vi "VI Tree.vi"   [LabVIEW 2012, in "Phidget Temperature Sensor.lvlib"]
doc: "${TemperatureSensor:VITreeHeader}"
uses:
  <instrlib>/Phidgets/Phidget Temperature Sensor/Phidget Temperature Sensor.lvlib
  <instrlib>/Phidgets/Phidget Temperature Sensor/Public/TemperatureSensorStart.vi
  <instrlib>/Phidgets/Phidget Temperature Sensor/Public/TemperatureSensorOpen.vi
  <instrlib>/Phidgets/Phidget Temperature Sensor/Public/TemperatureSensorClose.vi
panel:
  # "(c) 2015 Phidgets Inc..  ALL RIGHTS RESERVED."
  # "SEE DIAGRAM\nFOR VI TREE."
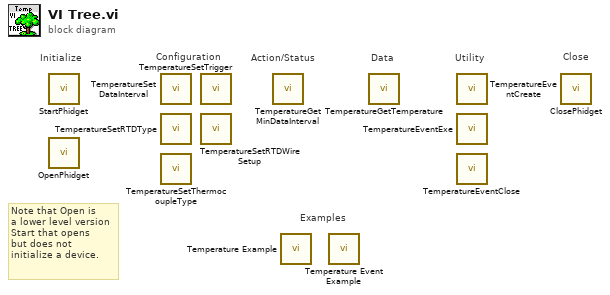
[diagram p0: block diagram]
diagram:
  # "Note that Open is\na lower level version\nStart that opens\nbut does not \ninitialize a device."
  # "Examples"
  # "Configuration"
  # "Utility"
  # "Data"
  # "Action/Status"
  # "Close"
  # "Initialize"
  n1 = call-poly <instrlib>:"StartPhidget.vi"() -> ()  [unwired: 12 in, 4 out]
  n2 = call-poly <instrlib>:"OpenPhidget.vi"() -> ()  [unwired: 8 in, 4 out]
  n3 = call <instrlib>:"TemperatureSetDataInterval.vi"() -> ()  [unwired: 9 in, 2 out]
  n4 = call <instrlib>:"TemperatureSetRTDType.vi"() -> ()  [unwired: 9 in, 2 out]
  n5 = call <instrlib>:"TemperatureSetThermocoupleType.vi"() -> ()  [unwired: 9 in, 2 out]
  n6 = call <instrlib>:"TemperatureSetTrigger.vi"() -> ()  [unwired: 9 in, 2 out]
  n7 = call <instrlib>:"TemperatureSetRTDWireSetup.vi"() -> ()  [unwired: 9 in, 2 out]
  n8 = call <instrlib>:"TemperatureGetMinDataInterval.vi"() -> ()  [unwired: 8 in, 3 out]
  n9 = call <instrlib>:"Temperature Example.vi"() -> ()  [unwired: 12 in]
  n10 = call <instrlib>:"Temperature Event Example.vi"() -> ()  [unwired: 12 in]
  n11 = call <instrlib>:"TemperatureGetTemperature.vi"() -> ()  [unwired: 8 in, 3 out]
  n12 = call <instrlib>:"TemperatureEventCreate.vi"() -> ()  [unwired: 9 in, 3 out]
  n13 = call <instrlib>:"TemperatureEventExe.vi"() -> ()  [unwired: 6 in, 6 out]
  n14 = call <instrlib>:"TemperatureEventClose.vi"() -> ()  [unwired: 10 in, 2 out]
  n15 = call-poly <instrlib>:"ClosePhidget.vi"() -> ()  [unwired: 11 in, 1 out]
